vi "test_Set-Get Protocol ConvBox.vi"(8 "error in (no error)":errorcluster, 11 "TestCase in":refnum<class "Instrument Addon Scripting API Custom Device Unit Tests.lvclass">) -> (0 "error out":errorcluster, 3 "TestCase out":refnum<class "Instrument Addon Scripting API Custom Device Unit Tests.lvclass">)   [LabVIEW 2018, in "Instrument Addon Scripting API Custom Device Unit Tests.lvclass"]
uses:
  Instrument Addon Scripting API Custom Device Unit Tests.lvclass
  Addon/Support Libraries/Protocols.lvlibp/RS-xxx to GPIB ConvBox/RS-xxx to GPIB ConvBox.lvclass
  D:/GitRepository/niveristand-instrument-addon-custom-device/Source/Addon/Support Libraries/Protocols.lvlibp/Protocol Parent/Protocol Parent.lvclass
  Addon/Support Libraries/Protocols.lvlibp/AK RS-xxx/AK RS-xxx.lvclass
  Instrument Addon Scripting API Custom Device Unit Tests.lvclass/Instrument Addon Scripting API Custom Device Unit Tests.ctl
  Addon/Support Libraries/Protocols.lvlibp/RS-xxx to GPIB ConvBox/Data Access/Write Assert Ren with IFC.vi
  Addon/Support Libraries/Protocols.lvlibp/RS-xxx to GPIB ConvBox/Data Access/Write ConvBox Address.vi
  Addon/Support Libraries/Protocols.lvlibp/RS-xxx to GPIB ConvBox/Data Access/Write GPIB Address.vi
  Addon/Support Libraries/Protocols.lvlibp/RS-xxx to GPIB ConvBox/Data Access/Write IST bit sense.vi
  Addon/Support Libraries/Protocols.lvlibp/RS-xxx to GPIB ConvBox/Data Access/Write Port.vi
  Addon/Support Libraries/Protocols.lvlibp/RS-xxx to GPIB ConvBox/Data Access/Write System controller.vi
  Instrument Addon Scripting API Test Assets/Instrument Addon Scripting API Test Assets.lvclass
  <vilib>/addons/_JKI Toolkits/VI Tester/TestCase.llb/TestCase.lvclass
  APIs/Scripting API/Instrument Addon Scripting API.lvlib
  C:/Program Files (x86)/National Instruments/LabVIEW 2018/vi.lib/addons/_JKI Toolkits/VI Tester/TestCase.llb/TestCase.lvclass
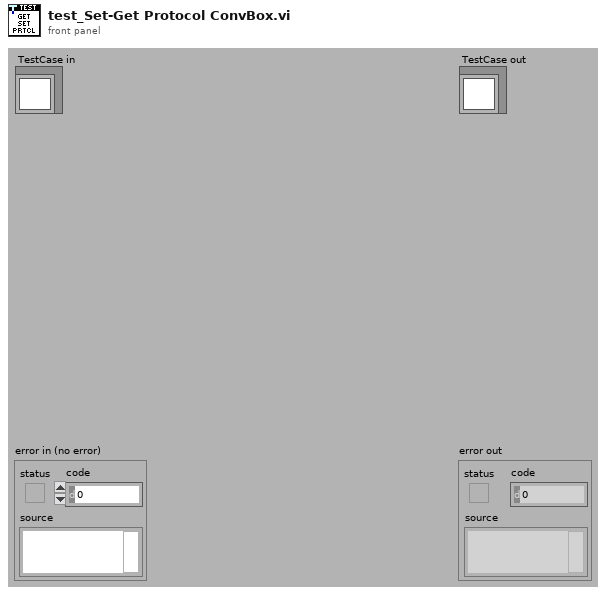
[diagram p1: front panel]
types:
  T1 = typedef "Custom Device API.lvlib/Custom Device Item Ref.ctl" = u64
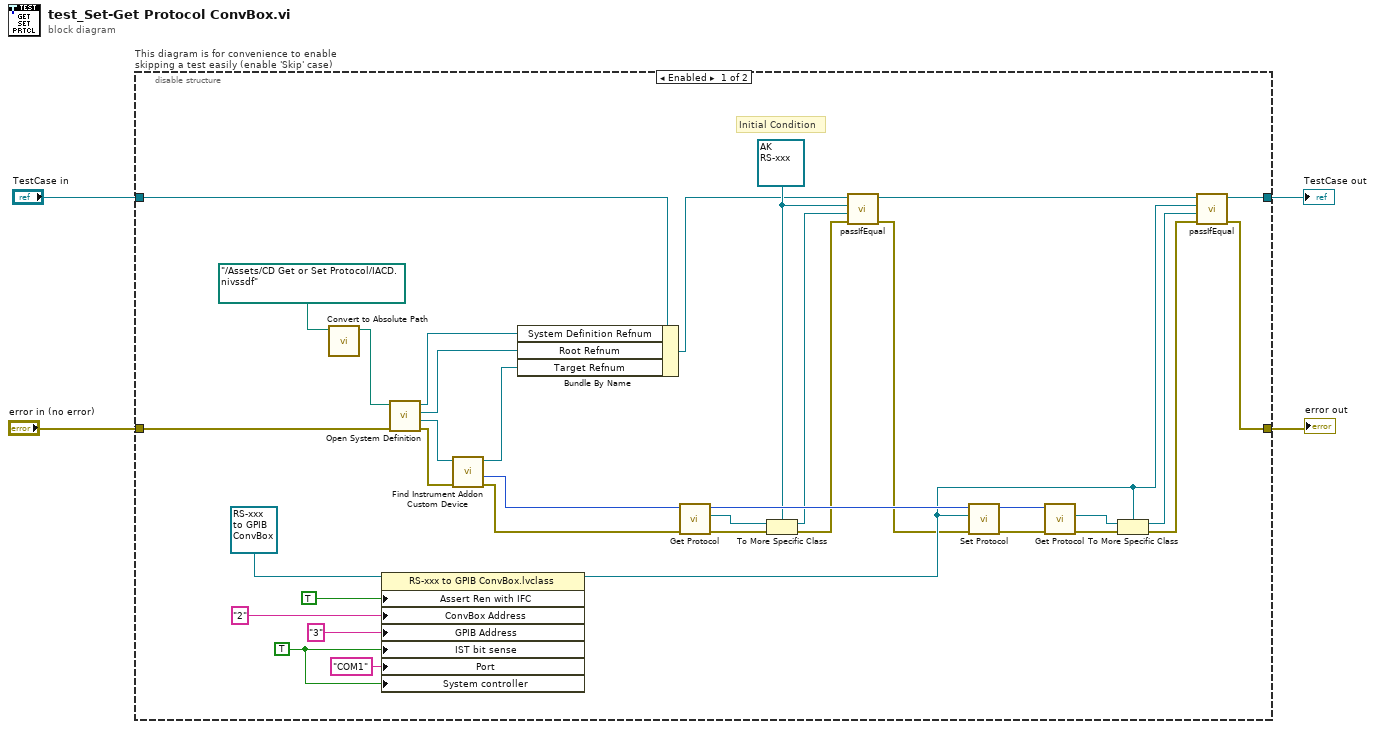
[diagram p0: block diagram]
diagram:
  n1 = disable-structure "This diagram is for convenience to enable skipping a test easily (enable 'Skip' case)" shown="Enabled" {
    disable-tunnel: "TestCase in" -> [w9 w43]
    disable-tunnel: [w29 w41] -> w1
    disable-tunnel: [w27 w42] -> w3
    disable-tunnel: "error in (no error)" -> [w39 w40]
    frame Enabled {
      w13 = refnum<class "AK RS-xxx.lvclass"> refnum ("reference out")
      w21 = TRUE ("Assert Ren with IFC")
      # "Initial Condition"
      n2 = call "Convert to Absolute Path.vi"("System Definition File"=path "../Assets/CD Get or Set Protocol/IACD.nivssdf" ("SDF file")) -> ("Absolute Path"=w37:path)  [unwired: 10 in]
      n3 = property class="RS-xxx to GPIB ConvBox.lvclass"(reference=refnum<class "RS-xxx to GPIB ConvBox.lvclass"> refnum ("Protocols.lvlibp:RS-xxx to GPIB ConvBox.lvclass"), "Assert Ren with IFC"=TRUE, "ConvBox Address"="2", "GPIB Address"="3" ("ConvBox Address"), "IST bit sense"=w21, "Port"="COM1", "System controller"=w21) -> (reference out=w14:refnum<class "RS-xxx to GPIB ConvBox.lvclass">)  [unwired: 1 in, 1 out]
      n4 = call "Open System Definition.vi"("error in (no error)"=w39, "System Definition File"=w37) -> ("error out"=w36:errorcluster, "Target Refnum"=w35:refnum<k24>, "Root Refnum"=w7:refnum<k24>, "System Definition Refnum"=w8:refnum<k24>)  [unwired: 6 in]
      n5 = call "Find Instrument Addon Custom Device.vi"("error in"=w36, "target in"=w35) -> ("error out"=w19:errorcluster, "NodeID"=w18:u64, "target out"=w6:refnum<k24>)  [unwired: 7 in]
      n6 = Bundle By Name(cluster=w9, "System Definition Refnum"=w8, "Root Refnum"=w7, "Target Refnum"=w6) -> (w5:refnum<class "Instrument Addon Scripting API Custom Device Unit Tests.lvclass">)
      n7 = call "Get Protocol.vi"("Error In"=w19, "Instrument Addon Refnum In"=w18) -> ("Error Out"=w15:errorcluster, "Protocol"=w20:refnum<class "Protocol Parent.lvclass">, "Instrument Addon Refnum Out"=w16:T1)  [unwired: 7 in]
      n8 = To More Specific Class(target class=w13, reference=w20, error in=w15) -> (specific class reference=w12:refnum<class "AK RS-xxx.lvclass">, error out=w11:errorcluster)
      n9 = call-dynamic "passIfEqual.vi"("error in (no error)"=w11, "y"=w12, "x"=w13, "TestCase in"=w5) -> ("error out"=w10:errorcluster, "TestCase out"=w17:refnum<class "Instrument Addon Scripting API Custom Device Unit Tests.lvclass">)  [unwired: 6 in]
      n10 = call "Set Protocol.vi"("Error In"=w10, "Protocol in"=w14, "Instrument Addon Refnum In"=w16) -> ("Error Out"=w33:errorcluster, "Instrument Addon Refnum Out"=w34:T1)  [unwired: 7 in]
      n11 = call "Get Protocol.vi"("Error In"=w33, "Instrument Addon Refnum In"=w34) -> ("Error Out"=w31:errorcluster, "Protocol"=w32:refnum<class "Protocol Parent.lvclass">)  [unwired: 7 in, 1 out]
      n12 = To More Specific Class(target class=w14, reference=w32, error in=w31) -> (specific class reference=w28:refnum<class "RS-xxx to GPIB ConvBox.lvclass">, error out=w30:errorcluster)
      n13 = call-dynamic "passIfEqual.vi"("error in (no error)"=w30, "y"=w28, "x"=w14, "TestCase in"=w17) -> ("error out"=w27:errorcluster, "TestCase out"=w29:refnum<class "Instrument Addon Scripting API Custom Device Unit Tests.lvclass">)  [unwired: 6 in]
    }
    frame Disabled {
      # "skip test result while test is under development"
      n14 = call <vilib>:"skip.vi"("error in (no error)"=w40, "TestCase in"=w43) -> ("error out"=w42:errorcluster, "TestCase out"=w41:refnum<class "Instrument Addon Scripting API Custom Device Unit Tests.lvclass">)  [unwired: 8 in]
    }
  }
  "error out" <- w3
  "TestCase out" <- w1
